vi "Close.vi"(8 "error in (no error)":errorcluster, 11 "Data in":refnum<class "Polled_EventSource.lvclass">) -> (0 "error out":errorcluster, 3 "Data out":refnum<class "Polled_EventSource.lvclass">)   [LabVIEW 2021, in "Polled_EventSource.lvclass"]
doc: "Abstract Data Classes 2.1.1.13\nTim Streeter - TSA\nCopyright (c) 2025, TSA"
uses:
  Polled_EventSource.lvclass
  <vilib>/TSA/Abstract Data Classes/Abs_Types/Value/Abs_Value.lvclass
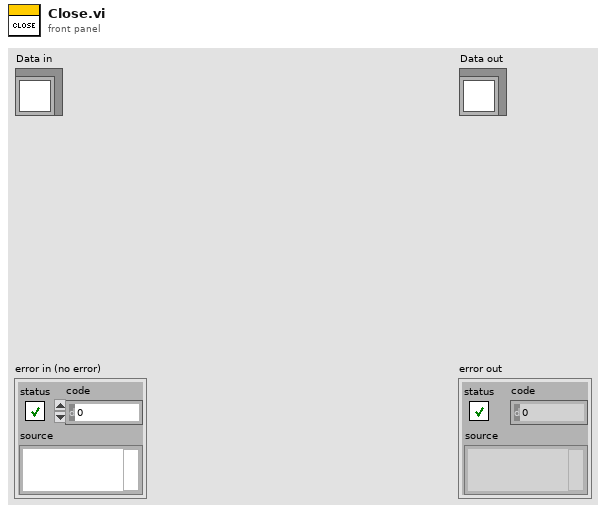
[diagram p1: front panel]
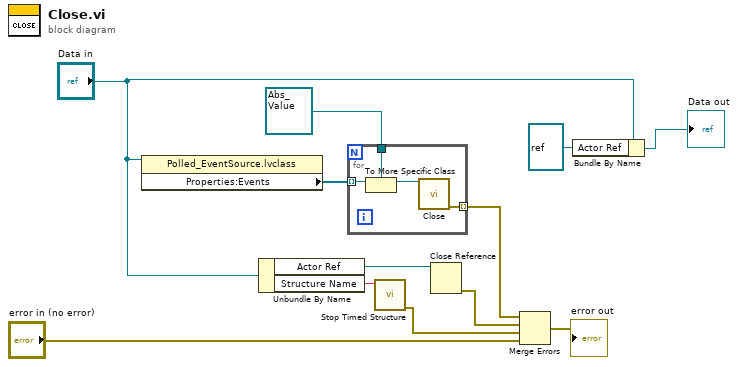
[diagram p0: block diagram]
diagram:
  n1 = property class="Polled_EventSource.lvclass"(reference="Data in") -> ("Properties:Events"=w3:refnum<class "Event_Polled Type.lvclass">[])  [unwired: 1 in, 2 out]
  n2 = Unbundle By Name("Data in") -> ("Actor Ref"=w10:refnum<vi>, "Structure Name"=w12:string)
  n3 = for {
    tunnel: w3 -> [w16] mode=indexing
    tunnel: refnum<class "Abs_Value.lvclass"> refnum ("Abs_Value.lvclass") -> [w14]
    tunnel: [w13] -> w1 mode=indexing
    n4 = To More Specific Class(target class=w14, reference=w16) -> (specific class reference=w15:refnum<class "Abs_Value.lvclass">)  [unwired: 1 in, 1 out]
    n5 = call-dynamic "Close.vi"("Data in"=w15) -> ("error out"=w13:errorcluster)  [unwired: 9 in, 1 out]
  }
  n6 = call <vilib>:"Stop Timed Structure.vi"("name"=w12) -> ("error out"=w11:errorcluster)  [unwired: 10 in]
  n7 = Close Reference(reference=w10) -> (error out=w9:errorcluster)  [unwired: 1 in]
  n8 = Merge Errors(w1, w9, w11, "error in (no error)") -> (→"error out":errorcluster)
  n9 = Bundle By Name(cluster="Data in", "Actor Ref"=refnum<vi> refnum) -> (→"Data out":refnum<class "Polled_EventSource.lvclass">)
